vi "RT_ReceiveRTNetworkStream.vi"(8 "ErrorIn":errorcluster, 10 "Reader in":refnum<k21>, 11 "queue":refnum<queue>) -> (0 "ErrorOut":errorcluster, 3 "endpoint out":refnum<k21>)   [LabVIEW 2018]
uses:
  Queue/RTMainQueueElements.ctl
  Controls/Clusts/StreamClust.ctl
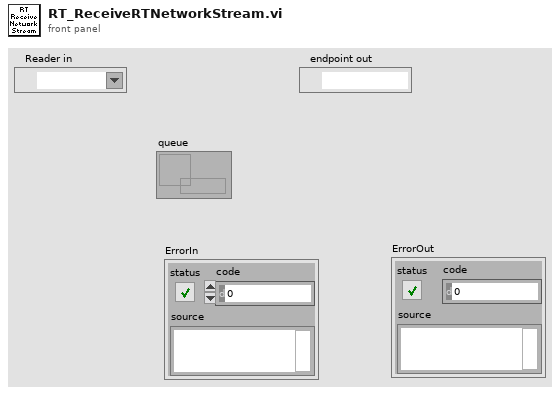
[diagram p1: front panel]
types:
  T1 = typedef "StreamClust.ctl" = cluster{u16, variant}
  T2 = typedef "RTMainQueueElements.ctl" = enum16{"RTMain_InitQ", "RTMain_InitSW", "RTMain_InitCtrls", "RTMain_ReInitHW", "RTMain_FromStream", "RTMain_StrtHWLp", "RTMain_UpdtHWClstr", "RTMain_Start", "RTMain_Stop", "RTMain_Error", "RTMain_Config", "RTMain_Exit"}
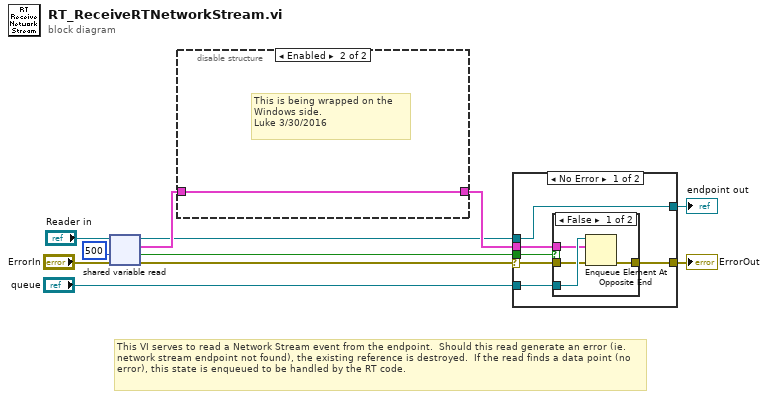
[diagram p0: block diagram]
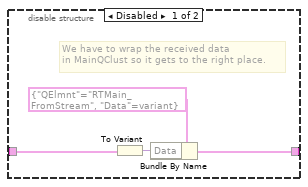
[diagram p2: hidden frame]
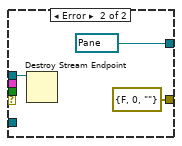
[diagram p4: hidden frame]
diagram:
  # "This VI serves to read a Network Stream event from the endpoint.  Should this read generate an error (ie. network stream endpoint not found), the existing reference is destroyed.  If the read finds a data point (no error), this state is enqueued to be handled by the RT code."
  n1 = shared-variable-read("Reader in", "ErrorIn", 500 ("Network Stream Polling Timeout (ms)")) -> (w2:refnum<k21>, w7:errorcluster, w10:bool, w5:T1)
  n2 = disable-structure shown="Enabled" {
    disable-tunnel: [w14 w16] -> w6
    disable-tunnel: w5 -> [w13 w16]
    frame Disabled {
      # "We have to wrap the received data\nin MainQClust so it gets to the right place."
      n3 = To Variant(anything=w13) -> (Variant=w15:variant)
      n4 = Bundle By Name(cluster=cluster{"QElmnt":T2, "Data":variant} {"QElmnt"=enum."RTMain_FromStream", "Data"=variant} ("Cluster"), "Data"=w15) -> (w14:cluster{"QElmnt":T2, "Data":variant})
    }
    frame Enabled {
      # "This is being wrapped on the \nWindows side.\nLuke 3/30/2016"
    }
  }
  n5 = case shown="No Error" w7 {
    selector: w7 -> [w20 _]
    tunnel: [w19 errorcluster {"status"=FALSE, "code"=0, "source"=""} ("error IO")] -> w11
    tunnel: w6 -> [w21 _]
    tunnel: w10 -> [w22 _]
    tunnel: w2 -> [w17 w30]
    tunnel: "queue" -> [w18 _]
    tunnel: [w17 refnum<k21> refnum ("endpoint out")] -> w1
    frame No Error {
      n6 = case shown="False" w22 {
        tunnel: w21 -> [w23 _]
        tunnel: w20 -> [w24 w27]
        tunnel: [w26 w27] -> w19
        tunnel: w18 -> [w25 _]
        frame False {
          n7 = Enqueue Element At Opposite End(queue=w25, element=w23, error in (no error)=w24) -> (error out=w26:errorcluster)  [unwired: 1 in, 2 out]
        }
        frame True {
        }
      }
    }
    frame Error {
      n8 = Destroy Stream Endpoint(11:w30) -> ()  [unwired: 1 in, 1 out]
    }
  }
  "ErrorOut" <- w11
  "endpoint out" <- w1
